vi "addArrayElement.vi"(7 "Name":string, 8 "error in (no error)":errorcluster, 9 "Value":refnum<class "tBSONElement.lvclass">[](array[class]), 10 "Replace? (false)":bool, 11 "tBSONDocument in":refnum<class "tBSONDocument.lvclass">) -> (0 "error out":errorcluster, 3 "tBSONDocument out":refnum<class "tBSONDocument.lvclass">)   [LabVIEW 2014, in "BSON.lvlib" / "tBSONDocument.lvclass"]
doc: "Adds an array of BSON elements to a BSON document."
uses:
  tBSONDocument.lvclass
  tBSONElement/tBSONElement.lvclass
  BSONElements/tBSONArray/tBSONArray.lvclass
  tBSONElement/setName.vi
  BSONElements/tBSONArray/setValue.vi
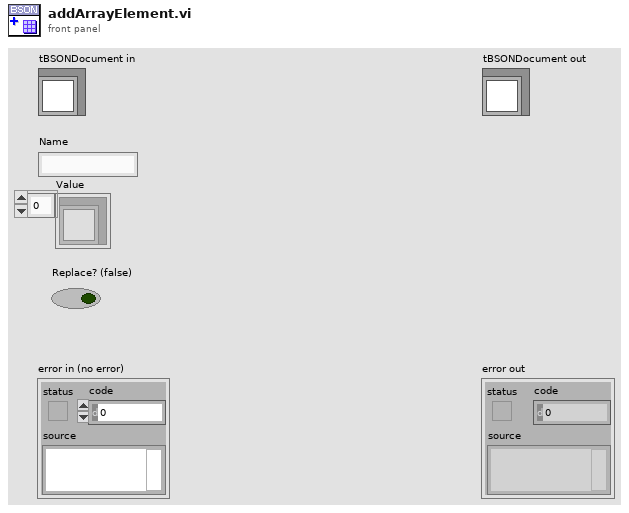
[diagram p1: front panel]
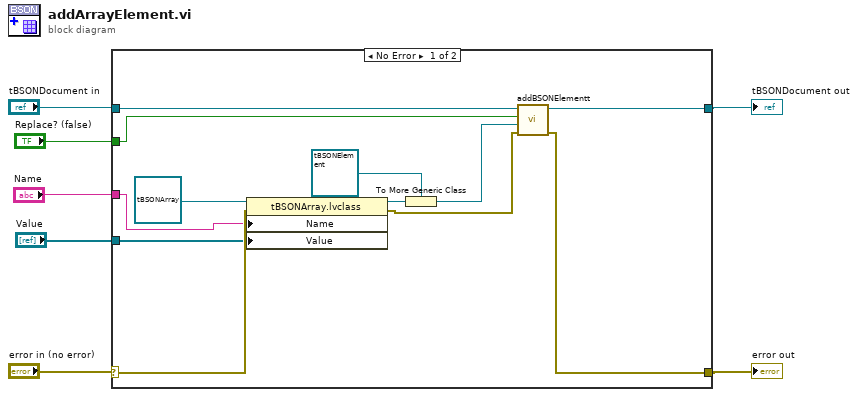
[diagram p0: block diagram]
diagram:
  n1 = case shown="No Error" "error in (no error)" {
    selector: "error in (no error)" -> [w19 w21]
    tunnel: [w13 w21] -> w4
    tunnel: [w15 w20] -> w6
    tunnel: "tBSONDocument in" -> [w16 w20]
    tunnel: "Name" -> [w11 _]
    tunnel: "Value" -> [w9 _]
    tunnel: "Replace? (false)" -> [w8 _]
    frame No Error {
      n2 = property class="tBSONArray.lvclass"(reference=refnum<class "tBSONArray.lvclass"> refnum ("BSON.lvlib:tBSONArray.lvclass"), error in=w19, "Name"=w11, "Value"=w9) -> (reference out=w18:refnum<class "tBSONArray.lvclass">, error out=w14:errorcluster)
      n3 = To More Generic Class(target class=refnum<class "tBSONElement.lvclass"> refnum ("BSON.lvlib:tBSONElement.lvclass"), reference=w18) -> (generic class reference=w12:refnum<class "tBSONElement.lvclass">)
      n4 = call "addBSONElementt.vi"("error in (no error)"=w14, "Element"=w12, "Replace? (false)"=w8, "tBSONDocument in"=w16) -> ("error out"=w13:errorcluster, "tBSONDocument out"=w15:refnum<class "tBSONDocument.lvclass">)  [unwired: 6 in]
    }
    frame Error {
    }
  }
  "error out" <- w4
  "tBSONDocument out" <- w6
